vi "week1Exercise2.vi"() -> ()   [LabVIEW 2015]
uses:
  <vilib>/LabVIEW Interface for Arduino/Type Defs/Board Type.ctl
  <vilib>/LabVIEW Interface for Arduino/Type Defs/Connection Type.ctl
  <vilib>/LabVIEW Interface for Arduino/LabVIEW Interface for Arduino.lvlib
panel:
  in  "Duty Cycle (0 - 255)":u8
  in  "stop":bool
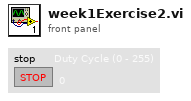
[diagram p1: front panel]
types:
  T1 = typedef "LabVIEW Interface for Arduino.lvlib/Connection Type.ctl" = enum8{"USB / Serial", "XBEE", "BlueSmirf (Bluetooth)"}
  T2 = typedef "LabVIEW Interface for Arduino.lvlib/Board Type.ctl" = enum16{"Uno", "Dimuelanove w/Atmega 328", "Mega 2560"}
  T3 = typedef "LabVIEW Interface for Arduino.lvlib/Arduino Resource.ctl" = cluster{"VISA resource":refnum<visa-resource-name>, "Board Type":T2, "Connection Type":enum8{"USB / Serial"}, "Bytes Per Packet (15)":u8}
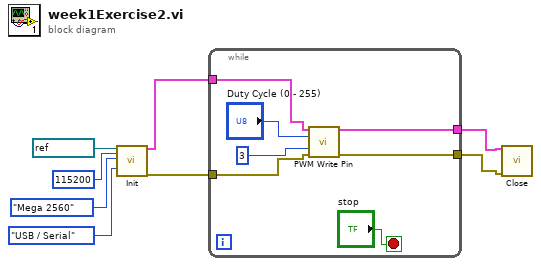
[diagram p0: block diagram]
diagram:
  n1 = call <vilib>:"Init.vi"("VISA resource"=refnum<visa-resource-name> "COM7", "Baud Rate (115200)"=u32 115200, "Board Type (Uno)"=Board_Type."Mega 2560", "Connection Type (USB/Serial)"=Connection_Type."USB / Serial") -> ("Arduino Resource"=w3:T3, "error out"=w4:errorcluster)  [unwired: 14 in]
  n2 = while {
    tunnel: w4 -> [w13]
    tunnel: w3 -> [w14]
    tunnel: [w12] -> w1
    tunnel: [w11] -> w2
    stop <- "stop" stop-if-true
    n3 = call <vilib>:"PWM Write Pin.vi"("Arduino Resource"=w14, "Duty Cycle (0 - 255)"="Duty Cycle (0 - 255)", "PWM Pin (3)"=u8 3, "error in"=w13) -> ("Arduino Resource"=w11:T3, "error out"=w12:errorcluster)  [unwired: 10 in]
  }
  n4 = call <vilib>:"Close.vi"("Arduino Resource"=w2, "error in"=w1) -> ()  [unwired: 13 in, 1 out]
